vi "Measure Thickness.vi"(8 "peak detector width":i32=3 min=3, 9 "threshold":dbl format="%0.2f", 11 "Input Array":dbl[][](array[numeric])) -> (0 "Amplitudes":dbl[](array[numeric]), 1 "peaks found":i32, 2 "Locations":dbl[](array[numeric]), 3 "uncorrected thickness":dbl)   [LabVIEW 2018]
uses:
  <vilib>/Analysis/NI_AAL_SigProc.lvlib
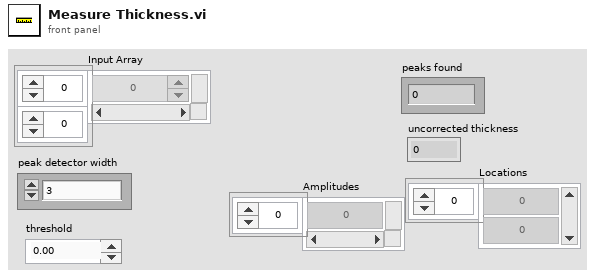
[diagram p1: front panel]
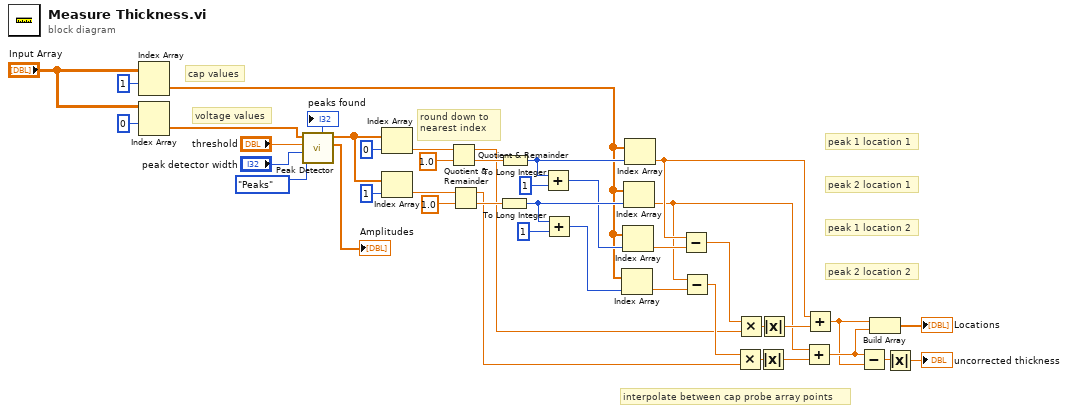
[diagram p0: block diagram]
diagram:
  # "voltage values"
  # "cap values"
  # "interpolate between cap probe array points"
  # "peak 2 location 2"
  # "peak 1 location 2"
  # "peak 2 location 1"
  # "peak 1 location 1"
  # "round down to\nnearest index"
  n1 = Index Array(array="Input Array", index (row)=1) -> (element=w18:dbl[])  [unwired: 1 in]
  n2 = Index Array(array="Input Array", index (row)=0) -> (element=w35:dbl[])  [unwired: 1 in]
  n3 = call <vilib>:"Peak Detector.vi"("peaks/valleys"=enum32{"Peaks", "Valleys"}."Peaks", "width"="peak detector width", "threshold"="threshold", "X"=w35) -> ("Amplitudes"=→"Amplitudes":dbl[], "Locations"=w30:dbl[], "# found"=→"peaks found":i32)  [unwired: 3 in, 2 out]
  n4 = Index Array(array=w30, index=0) -> (element=w28:dbl)
  n5 = Index Array(array=w30, index=1) -> (element=w25:dbl)
  n6 = Quotient & Remainder(x=w28, y=1.0) -> (x-y*floor(x/y)=w4:dbl, floor(x/y)=w11:dbl)
  n7 = Quotient & Remainder(x=w25, y=1.0) -> (x-y*floor(x/y)=w3:dbl, floor(x/y)=w10:dbl)
  n8 = To Long Integer(number=w10) -> (32bit integer=w24:i32)
  n9 = To Long Integer(number=w11) -> (32bit integer=w23:i32)
  n10 = Add(x=w23, y=1) -> (x+y=w20:i32)
  n11 = Add(x=w24, y=1) -> (x+y=w19:i32)
  n12 = Index Array(array=w18, index=w19) -> (element=w16:dbl)
  n13 = Index Array(array=w18, index=w20) -> (element=w17:dbl)
  n14 = Index Array(array=w18, index=w24) -> (element=w6:dbl)
  n15 = Index Array(array=w18, index=w23) -> (element=w7:dbl)
  n16 = Subtract(x=w7, y=w17) -> (x-y=w15:dbl)
  n17 = Subtract(x=w6, y=w16) -> (x-y=w14:dbl)
  n18 = Multiply(x=w14, y=w3) -> (x*y=w12:dbl)
  n19 = Multiply(x=w15, y=w4) -> (x*y=w13:dbl)
  n20 = Absolute Value(x=w12) -> (abs(x)=w8:dbl)
  n21 = Absolute Value(x=w13) -> (abs(x)=w9:dbl)
  n22 = Add(x=w6, y=w8) -> (x+y=w2:dbl)
  n23 = Add(x=w7, y=w9) -> (x+y=w1:dbl)
  n24 = Subtract(x=w2, y=w1) -> (x-y=w32:dbl)
  n25 = Build Array(w1, w2) -> (→"Locations":dbl[])
  n26 = Absolute Value(x=w32) -> (abs(x)=→"uncorrected thickness":dbl)
